vi "DSF.Engine.Transceiver Loader.Find Classes.vi"(8 "error in (no error)":errorcluster, 11 "Transceiver Loader in":refnum<class "DSF.Engine.Transceiver Loader.lvclass">) -> (0 "error out":errorcluster, 2 "class paths":path[](array[path]), 3 "Transceiver Loader out":refnum<class "DSF.Engine.Transceiver Loader.lvclass">)   [LabVIEW 2017, in "Data Sharing Framework Engine.lvlib" / "DSF.Engine.Transceiver Loader.lvclass"]
uses:
  DSF.Engine.Transceiver Loader.lvclass
  <vilib>/Utility/LVLibp/NI_PackedLibraryUtility.lvlib
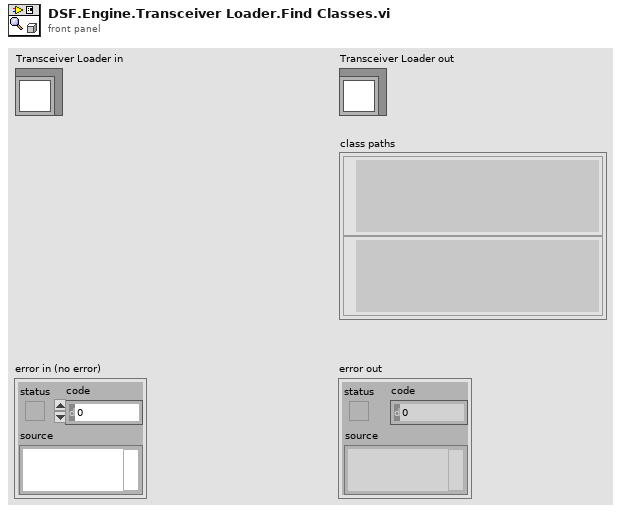
[diagram p1: front panel]
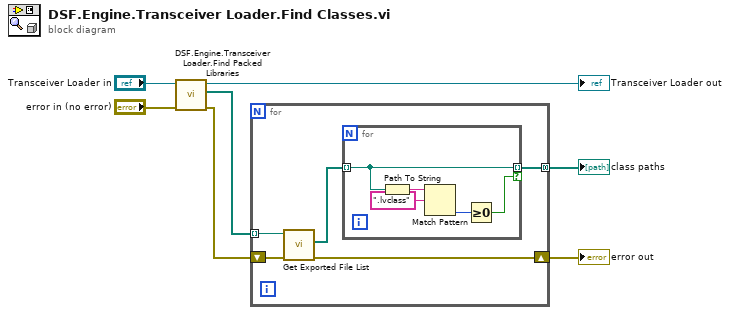
[diagram p0: block diagram]
diagram:
  n1 = call "DSF.Engine.Transceiver Loader.Find Packed Libraries.vi"("error in (no error)"="error in (no error)", "Transceiver Loader in"="Transceiver Loader in") -> ("error out"=w5:errorcluster, "packed library paths"=w1:path[], "Transceiver Loader out"=→"Transceiver Loader out":refnum<class "DSF.Engine.Transceiver Loader.lvclass">)  [unwired: 7 in]
  n2 = for {
    tunnel: w1 -> [w11] mode=indexing
    shift-right: [w9] -> w3
    shift-left: w5 -> [w10]
    tunnel: [w8] -> w2 mode=concatenating
    n3 = call <vilib>:"Get Exported File List.vi"("error in (no error)"=w10, "packed library path"=w11) -> ("error out"=w9:errorcluster, "paths"=w12:path[])  [unwired: 7 in, 1 out]
    n4 = for {
      tunnel: w12 -> [w15] mode=indexing
      tunnel: [w15] -> w8 mode=indexing if=w13
      n5 = Path To String(path=w15) -> (string=w16:string)
      n6 = Match Pattern(string=w16, regular expression=".lvclass") -> (offset past match=w14:i32)  [unwired: 1 in, 3 out]
      n7 = Greater Or Equal To 0?(x=w14) -> (x >= 0?=w13:bool)
    }
  }
  "error out" <- w3
  "class paths" <- w2
